vi "Initialise.vi"(8 "error in (no error)":errorcluster, 11 "Max Steps (10)":i32=10) -> (0 "error out":errorcluster, 3 "Sequencer out":refnum<class "Sequencer.lvclass">)   [LabVIEW 2020, in "Sequencer.lvclass"]
uses:
  Sequencer.lvclass
  Single Step Data.ctl
  Sequencer.lvclass/Sequencer.ctl
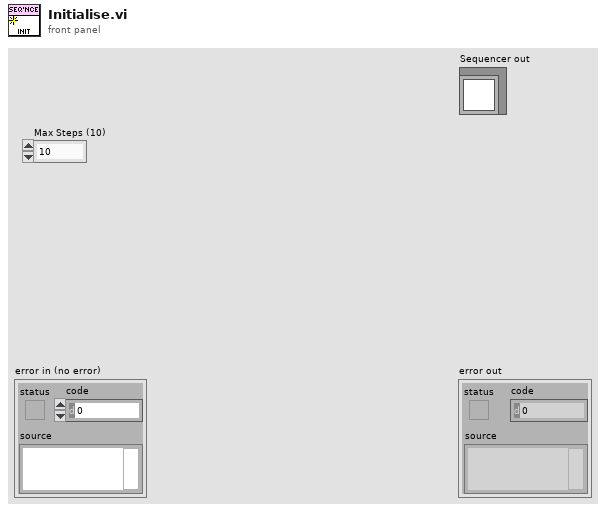
[diagram p1: front panel]
types:
  T1 = typedef "Sequencer.lvclass/Single Step Data.ctl" = cluster{"Name":string, "Parameter":variant, "Reply Channel":refnum<notifier>}
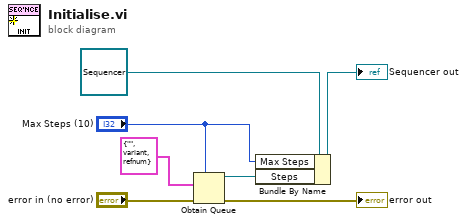
[diagram p0: block diagram]
diagram:
  n1 = Obtain Queue(max queue size (-1, unlimited)="Max Steps (10)", element data type=T1 {"Name"="", "Parameter"=variant, "Reply Channel"=refnum} ("Cluster"), error in (no error)="error in (no error)") -> (queue out=w3:refnum<queue>, error out=→"error out":errorcluster)  [unwired: 2 in, 1 out]
  n2 = Bundle By Name(cluster=refnum<class "Sequencer.lvclass"> refnum ("Sequencer in"), "Max Steps"="Max Steps (10)", "Steps"=w3) -> (→"Sequencer out":refnum<class "Sequencer.lvclass">)
